vi "ParseIssueNumber.vi"(1 "String":string) -> (0 "Numeric":dbl)   [LabVIEW 2024]
uses:
  <userlib>/_OpenG.lib/file/file.llb/openg_file.lvlib
  <userlib>/_OpenG.lib/file/file.llb/Strip Path Extension - String__ogtk.vi
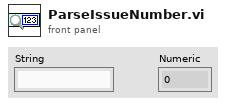
[diagram p1: front panel]
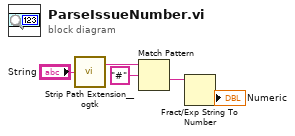
[diagram p0: block diagram]
diagram:
  n1 = call-poly <userlib>:"Strip Path Extension__ogtk.vi"("path"="String") -> ("root"=w2:string)  [unwired: 1 out]
  n2 = Match Pattern(string=w2, regular expression="#") -> (after substring=w4:string)  [unwired: 1 in, 3 out]
  n3 = Fract/Exp String To Number(string=w4) -> (number=→"Numeric":dbl)  [unwired: 3 in, 1 out]
